vi "Diagnostics.Main.vi"(8 "error in (no error)":errorcluster, 11 "State Variables":T1={"TCP Refs"={"Connection List"=refnum, "listener ID"=refnum}, "Stop"=refnum, "Top VI"=refnum, "Parameters"={"Properties"={"Name"="", "CAN"={"CAN Interface"=enum."CAN0", "Baud Rate"=0, "Diagnostic Protocol"=enum."GMLAN", "Transport Protocol"=enum."ISO TP - Normal Mode", "Transmit ID"=0, "Receive ID"=0, "Transmit Extension"=0, "Receive Extension"=0, "Receive UUDT ID"=0, "Enable Stream"=TRUE, "VW TP Channel ID"=0, "Security"={"Source DLL Path"=path "", "Security Level"=1, "Target DLL Path"=path ""}, "Fill Frame"=FALSE, "Fill Byte"=255, "Termination"=FALSE}, "986x"={"Enable"=FALSE, "RIO Device"=0, "Bitfile"=path ""}, "Reads"=[], "Frames Lookup"=variant, "Writes"=[], "DPIDs"=[], "DPID Lookup"=variant, "DTC descriptor"={"DTC Byte Length"=2, "Status Byte Length"=1, "Add Data Byte Length"=1, "Byte Order"=enum."Motorola"}}, "ChanRefs"={"ToVS.Reads"={"Name"="", "Write to VS Engine FIFO"=refnum, "Pairs"={"Refs"=[], "Values"=[]}}, "ToVS.DTCs"={"Name"="", "Write to VS Engine FIFO"=refnum, "Pairs"={"Refs"=[], "Values"=[]}}, "ToVS.DTCCount"={"Name"="", "Write to VS Engine FIFO"=refnum, "Pairs"={"Refs"=[], "Values"=[]}}, "ToVS.Status"={"Name"="", "Write to VS Engine FIFO"=refnum, "Pairs"={"Refs"=[], "Values"=[]}}, "FromVS.Writes"={"Name"="", "Read from VS Engine FIFO"=refnum, "Pairs"={"Refs"=[], "Values"=[]}}, "Cmds"={"Name"="", "Write to VS Engine FIFO"=refnum, "Read from VS Engine FIFO"=refnum, "Pairs"={"Chan Refs"=[], "Prev. Values"=[]}}}}, "ADCS Connection"={"Diag CAN Handle"=0, "Transport Protocol"=enum."ISO TP - Normal Mode", "Receive Address Extension"=0, "Transmit Address Extension"=0, "Receive CAN Id"=0, "Transmit CAN Id"=0, "Diag CAN Queue"=refnum, "Log Frames ?"=FALSE, "My TP Address"=0, "Other TP Address"=0, "T1"=0, "T2"=0, "T3"=0, "T4"=0, "Tx SN"=0, "Block Size"=0, "Rx SN"=0, "VW TP Initialized?"=FALSE, "Tx block no"=0, "baud rate"=0, "Interface"="", "Channel Diag CAN Handle"=0, "UDP Connection ID"=refnum, "TCP Connection ID"=refnum, "Target IP Addr"=0, "Source Address"=0, "Target Address"=0, "Send Header NACK?"=FALSE, "DLL Handle"=0, "NAD"=0, "Time Stamp read first"=0.0, "Time Stamp read last"=0.0, "Time Stamp write first"=0.0, "Time Stamp write last"=0.0, "Time Stamp write"=0.0, "Time Stamp read"=0.0}, "XNET References"={"Database"="", "GMLAN DPID Session"="", "Cluster"=""}, "BufferedCmds"=refnum, "XNETEngine (GMLAN)"=refnum} {"Parameters"."ChanRefs"."Cmds"."Pairs"."Chan Refs" format="%.0x"; "Parameters"."ChanRefs"."ToVS.Status"."Pairs"."Refs" format="%.0x"; "Parameters"."ChanRefs"."ToVS.DTCCount"."Pairs"."Refs" format="%.0x"; "Parameters"."ChanRefs"."ToVS.DTCs"."Pairs"."Refs" format="%.0x"; "Parameters"."ChanRefs"."ToVS.Reads"."Pairs"."Refs" format="%.0x"; "Parameters"."Properties"."Writes"."Signals"."Byte Order" items=["Little Endian", "Big Endian"]; "Parameters"."Properties"."Writes"."Signals"."Data Type" items=["Signed", "Unsigned", "IEEE Float"]; "Parameters"."Properties"."CAN"."Fill Byte" format="%.0x"; "Parameters"."Properties"."CAN"."VW TP Channel ID" format="%.0x"; "Parameters"."Properties"."CAN"."Receive UUDT ID" format="%.0x"; "Parameters"."Properties"."CAN"."Receive Extension" format="%.0x"; "Parameters"."Properties"."CAN"."Transmit Extension" format="%.0x"; "Parameters"."Properties"."CAN"."Receive ID" format="%.0x"; "Parameters"."Properties"."CAN"."Transmit ID" format="%.0x"; "Parameters"."Properties"."Reads"."Signals"."Byte Order" items=["Little Endian", "Big Endian"]; "Parameters"."Properties"."Reads"."Signals"."Data Type" items=["Signed", "Unsigned", "IEEE Float"]}) -> (0 "error out":errorcluster)   [LabVIEW 2015, in "Diagnostics Addon Engine.lvlib"]
uses:
  Diagnostics Addon Engine.lvlib
  Types/Diagnostics.State.ctl
  Types/TCP.Refs.ctl
  STM/STM Lookup Table Ref.ctl
  Stop FG/Stop Global Ref.ctl
  Types/Engine.State.ctl
  Shared/Types/SysDef.Compile.Properties.ctl
  Shared/Types/CAN.ctl
  Shared/Types/CAN.Interface.ctl
  Shared/Types/Protocol.ctl
  Shared/Types/Transport.ctl
  Shared/Types/Security.ctl
  Shared/Types/986x.ctl
  Shared/Types/Frame.Compile.ctl
  Shared/Types/Type.ctl
  Shared/Types/Signal.ctl
  Shared/Types/DPID.ctl
  Shared/Types/DPID.Rate.ctl
  Shared/Types/DTCDescriptor.ctl
  Types/Engine.Refs.ctl
  Inline Async API/Controls/Write To VS Engine.ctl
  <vilib>/NI Veristand/Custom Device API/Data Reference.ctl
  Inline Async API/Controls/Read From VS Engine.ctl
  <vilib>/NI Veristand/Custom Device API/Block Data Reference.ctl
  Inline Async API/Controls/ReadWrite Data.ctl
  <vilib>/Automotive Diagnostic Command Set/Diagnostic Transport.llb/Diag Reference.ctl
  <vilib>/Automotive Diagnostic Command Set/Diagnostic Transport.llb/Transport Protocol Selector.ctl
  <vilib>/Automotive Diagnostic Command Set/Diagnostic Transport.llb/Diag CAN Frame Log.ctl
  Types/XNET.Refs.ctl
  <vilib>/NI/AMC/Message Queue.ctl
  <vilib>/NI/AMC/Message.ctl
  <vilib>/NI/Tools/Keyed Array/KeyedArray.ctl
  Stop FG/Global Stop Actions.vi
  Signals.Scale.EU.vi
  Frame.Build.Raw.vi
  <vilib>/NI/AMC/Send Local Message.vi
  GMLAN/Utilities/Convert Data to DTCs.vi
  DTCs.List.Update.vi
  <vilib>/NI/AMC/Read Next Message.vi
  GMLAN/_SubVIs/ReadDiagnosticInformation_ByStatus.vi
  Status.Set.vi
  GMLAN/_SubVIs/ReadDiagnosticInformation_sendOnChangeDTCCount.vi
  GMLAN/_SubVIs/ReadDiagnosticInformation_readStatusOfDTCByDTCNumber.vi
  GMLAN/_SubVIs/ReadFailureRecordData_readFailureRecordParameters.vi
  GMLAN/GMLAN DynamicallyDefineMessage.vi
  GMLAN/GMLAN ReadDataByPacketIdentifier.vi
  Signals.Scale.Raw.vi
  GMLAN/GMLAN DeviceControl.vi
  GMLAN/GMLAN TesterPresent.vi
  GMLAN/GMLAN InitiateDiagnosticOperation.vi
  GMLAN/GMLAN DisableNormalCommunication.vi
  GMLAN/GMLAN ReturnToNormalMode.vi
  ADCS.UnlockECUSecurity.vi
  <vilib>/NI/Tools/Keyed Array/Index.vi
  GMLAN/GMLAN ClearDiagnosticInformation.vi
  GMLAN/GMLAN ReadDataByParameterIdentifier.vi
  GMLAN/GMLAN ReadDataByIdentifier.vi
  Frames.Lookup.Size.Get.vi
  ADCS.TesterPresent.vi
  <vilib>/NI/AMC/Create Single Message.vi
  <vilib>/NI/AMC/Update Message Routing Info.vi
  GMLAN/Utilities/Convert Raw Data to DTCs.vi
  <vilib>/NI/AMC/Read Termination Message.vi
  <vilib>/Utility/error.llb/Clear Errors.vi
  ADCS.Get.ErrorByte.vi
  GMLAN/Utilities/GMLAN Service Broadcast.vi
  Security.DLL
  GMLAN/GMLAN SecurityAccess.vi
  GMLAN/_SubVIs/SecurityAccess_sendKey.vi
  GMLAN/_SubVIs/SecurityAccess_requestSeed.vi
  <vilib>/NI/Tools/Keyed Array/Map String.vi
  <vilib>/NI/Tools/String/Get Case Matching.vi
  Error Handling API/SubVIs/Report Error to Process.vi
  <vilib>/NI/AMC/Send Message.vi
  <vilib>/Automotive Diagnostic Command Set/Diagnostic Protocols.llb/Convert to Phys.vi
  <vilib>/xnet/xnet.llb/XNET Convert.vi
  <vilib>/xnet/xnet.llb/XNET Convert (Frame Raw to Signal).vi
  ID.Convert.Raw.vi
  <vilib>/NI Veristand/Custom Device Tools/Custom Device Utility Library/NI VeriStand - Print Debug String.vi
  <vilib>/xnet/xnet.llb/XNET Read.vi
  <vilib>/xnet/xnet.llb/XNET Read (Frame CAN).vi
  Shared/SubVIs/Constants.vi
  <vilib>/NI/AMC/Globals.vi
  <vilib>/Automotive Diagnostic Command Set/Diagnostic Protocols.llb/UDS TesterPresent.vi
  <vilib>/Automotive Diagnostic Command Set/Diagnostic Transport.llb/Apply Success Failure Error.vi
  <vilib>/Automotive Diagnostic Command Set/Diagnostic Transport.llb/Diagnostic Service.vi
  <vilib>/Automotive Diagnostic Command Set/Diagnostic Transport.llb/Apply Diagnostic Error.vi
  <vilib>/Automotive Diagnostic Command Set/Diagnostic Transport.llb/Diagnostic Response Recv.vi
  <vilib>/Automotive Diagnostic Command Set/Diagnostic Transport.llb/Diagnostic Service Send.vi
  <vilib>/Automotive Diagnostic Command Set/Diagnostic Transport.llb/Diag Globals.vi
  <vilib>/Automotive Diagnostic Command Set/Diagnostic Protocols.llb/TesterPresent.vi
  <vilib>/Automotive Diagnostic Command Set/Diagnostic Protocols.llb/UDS RoutineControl.vi
  <vilib>/Automotive Diagnostic Command Set/Diagnostic Protocols.llb/StopRoutineByLocalIdentifier.vi
  <vilib>/xnet/xnet.llb/XNET Convert (Signal to Frame Raw).vi
  <vilib>/Automotive Diagnostic Command Set/Diagnostic Protocols.llb/RequestRoutineResultsByLocalIdentifier.vi
  <vilib>/Automotive Diagnostic Command Set/Diagnostic Protocols.llb/StartRoutineByLocalIdentifier.vi
  <vilib>/Automotive Diagnostic Command Set/Diagnostic Protocols.llb/UDS InputOutputControlByIdentifier.vi
  <vilib>/Automotive Diagnostic Command Set/Diagnostic Protocols.llb/InputOutputControlByLocalIdentifier.vi
  <vilib>/Automotive Diagnostic Command Set/Diagnostic Protocols.llb/UDS WriteMemoryByAddress.vi
  <vilib>/Automotive Diagnostic Command Set/Diagnostic Protocols.llb/UDS06 WriteMemoryByAddress.vi
  <vilib>/Automotive Diagnostic Command Set/Diagnostic Protocols.llb/WriteMemoryByAddress.vi
  <vilib>/Automotive Diagnostic Command Set/Diagnostic Protocols.llb/UDS ReadMemoryByAddress.vi
  <vilib>/Automotive Diagnostic Command Set/Diagnostic Protocols.llb/UDS06 ReadMemoryByAddress.vi
  <vilib>/Automotive Diagnostic Command Set/Diagnostic Protocols.llb/ReadMemoryByAddress.vi
  <vilib>/Automotive Diagnostic Command Set/Diagnostic Protocols.llb/UDS ECUReset.vi
  <vilib>/Automotive Diagnostic Command Set/Diagnostic Protocols.llb/ECUReset.vi
  <vilib>/Automotive Diagnostic Command Set/Diagnostic Protocols.llb/ControlDTCSetting.vi
  <vilib>/Automotive Diagnostic Command Set/Diagnostic Protocols.llb/UDS ControlDTCSetting.vi
  <vilib>/Automotive Diagnostic Command Set/Diagnostic Protocols.llb/UDS WriteDataByIdentifier.vi
  <vilib>/Automotive Diagnostic Command Set/Diagnostic Protocols.llb/WriteDataByLocalIdentifier.vi
  <vilib>/Automotive Diagnostic Command Set/Diagnostic Protocols.llb/UDS ReadDataByIdentifier.vi
  <vilib>/Automotive Diagnostic Command Set/Diagnostic Protocols.llb/ReadDataByLocalIdentifier.vi
  <vilib>/Automotive Diagnostic Command Set/Diagnostic Protocols.llb/UDS ClearDiagnosticInformation.vi
  <vilib>/Automotive Diagnostic Command Set/Diagnostic Protocols.llb/ClearDiagnosticInformation.vi
  <vilib>/Automotive Diagnostic Command Set/Diagnostic Protocols.llb/ReadDTCByStatus.vi
  <vilib>/Automotive Diagnostic Command Set/Diagnostic Protocols.llb/ReadStatusOfDTC.vi
  <vilib>/Automotive Diagnostic Command Set/Diagnostic Protocols.llb/UDS ReportDTCByStatusMask.vi
  <vilib>/Automotive Diagnostic Command Set/Diagnostic Protocols.llb/UDS ReportSeverityInformationOfDTC.vi
  <vilib>/Automotive Diagnostic Command Set/Diagnostic Protocols.llb/UDS ReportDTCBySeverityMaskRecord.vi
  <vilib>/Automotive Diagnostic Command Set/Diagnostic Protocols.llb/SendKey.vi
  <vilib>/Automotive Diagnostic Command Set/Diagnostic Protocols.llb/UDS SendKey.vi
  <vilib>/Automotive Diagnostic Command Set/Diagnostic Protocols.llb/RequestSeed.vi
  <vilib>/Automotive Diagnostic Command Set/Diagnostic Protocols.llb/UDS RequestSeed.vi
  <vilib>/Automotive Diagnostic Command Set/Diagnostic Protocols.llb/EnableNormalMessageTransmission.vi
  <vilib>/Automotive Diagnostic Command Set/Diagnostic Protocols.llb/UDS CommunicationControl.vi
  <vilib>/Automotive Diagnostic Command Set/Diagnostic Protocols.llb/DisableNormalMessageTransmission.vi
  <vilib>/Automotive Diagnostic Command Set/Diagnostic Protocols.llb/UDS DiagnosticSessionControl.vi
  <vilib>/Automotive Diagnostic Command Set/Diagnostic Protocols.llb/StopDiagnosticSession.vi
  <vilib>/Automotive Diagnostic Command Set/Diagnostic Protocols.llb/StartDiagnosticSession.vi
  <vilib>/Automotive Diagnostic Command Set/Diagnostic Transport.llb/Diag Set Property.vi
  <vilib>/Automotive Diagnostic Command Set/Diagnostic Transport.llb/Diag Get Property.vi
  DPIDs.IDs.Sort.vi
  Shared/Diagnostics Addon Shared.lvlib
  <vilib>/NI Veristand/Custom Device API/Custom Device API.lvlib
  <vilib>/NI/Tools/Keyed Array/Tools_KeyedArray.lvlib
  <vilib>/NI/AMC/AMC.lvlib
  <vilib>/addons/Automotive Diagnostic Command Set/NI_Automotive Diagnostic Command Set.lvlib
  Inline Async API/Inline Async API.lvlib
  Stop FG/Stop FG.lvlib
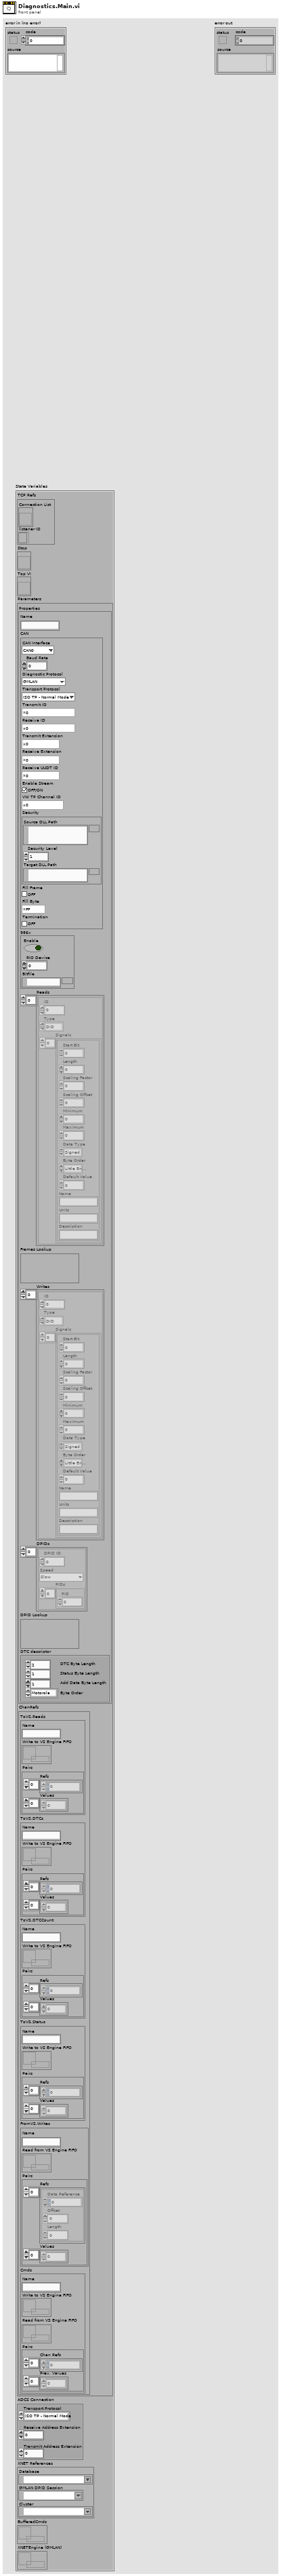
[diagram p1: front panel]
types:
  T1 = typedef "Diagnostics Addon Engine.lvlib/Diagnostics.State.ctl" = cluster{"TCP Refs":T2, "Stop":T4, "Top VI":refnum<vi>, "Parameters":T5, "ADCS Connection":T25, "XNET References":T27, "BufferedCmds":T28, "XNETEngine (GMLAN)":T28}
  T2 = typedef "Diagnostics Addon Engine.lvlib/TCP.Refs.ctl" = cluster{"Connection List":T3, "listener ID":refnum<k5>}
  T3 = typedef "Diagnostics Addon Engine.lvlib/STM Lookup Table Ref.ctl" = refnum<vi>
  T4 = typedef "Diagnostics Addon Engine.lvlib/Stop FG.lvlib/Stop Global Ref.ctl" = refnum<vi>
  T5 = typedef "Diagnostics Addon Engine.lvlib/Engine.State.ctl" = cluster{"Properties":T6, "ChanRefs":T19}
  T6 = typedef "Diagnostics Addon Shared.lvlib/SysDef.Compile.Properties.ctl" = cluster{"Name":string, "CAN":T7, "986x":T12, "Reads":T13[], "Frames Lookup":variant, "Writes":T13[], "DPIDs":T16[], "DPID Lookup":variant, "DTC descriptor":T18}
  T7 = typedef "Diagnostics Addon Shared.lvlib/CAN.ctl" = cluster{"CAN Interface":T8, "Baud Rate":u32, "Diagnostic Protocol":T9, "Transport Protocol":T10, "Transmit ID":u32, "Receive ID":u32, "Transmit Extension":u8, "Receive Extension":u8, "Receive UUDT ID":u32, "Enable Stream":bool, "VW TP Channel ID":u32, "Security":T11, "Fill Frame":bool, "Fill Byte":u8, "Termination":bool}
  T8 = typedef "Diagnostics Addon Shared.lvlib/CAN.Interface.ctl" = enum16{"CAN0", "CAN1", "CAN2", "CAN3", "CAN4", "CAN5", "CAN6", "CAN7", "CAN8", "CAN9", "CAN10", "CAN11", "CAN12", "CAN13", "CAN14", "CAN15", "CAN16", "CAN17", "CAN18", "CAN19", "CAN20", "CAN21", "CAN22", "CAN23", "CAN24", "CAN25", "CAN26", "CAN27", "CAN28", "CAN29", "CAN30", "CAN31", "CAN32", "CAN33", "CAN34", "CAN35", "CAN36", "CAN37", "CAN38", "CAN39", "CAN40", "CAN41", "CAN42", "CAN43", "CAN44", "CAN45", "CAN46", "CAN47", "CAN48", "CAN49", "CAN50", "CAN51", "CAN52", "CAN53", "CAN54", "CAN55", "CAN56", "CAN57", "CAN58", "CAN59", "CAN60", "CAN61", "CAN62", "CAN63", "CAN 256 (Virtual)", "CAN 257 (Virtual)"}
  T9 = typedef "Diagnostics Addon Shared.lvlib/Protocol.ctl" = enum16{"GMLAN", "KWP-2000", "UDS"}
  T10 = typedef "Diagnostics Addon Shared.lvlib/Transport.ctl" = enum16{"ISO TP - Normal Mode", "ISO TP - Mixed Mode", "VW TP 2.0", "Diagnostics on IP"}
  T11 = typedef "Diagnostics Addon Shared.lvlib/Security.ctl" = cluster{"Source DLL Path":path, "Security Level":u8, "Target DLL Path":path}
  T12 = typedef "Diagnostics Addon Shared.lvlib/986x.ctl" = cluster{"Enable":bool, "RIO Device":u16, "Bitfile":path}
  T13 = typedef "Diagnostics Addon Shared.lvlib/Frame.Compile.ctl" = cluster{"ID":u32, "Type":T14, "Signals":T15[]}
  T14 = typedef "Diagnostics Addon Shared.lvlib/Type.ctl" = enum16{"DID", "CDID", "PID", "CPID", "Read Memory", "Write Memory", "DTC Control", "IO Cmd", "IO Resp", "Routine Start Cmd", "Routine Start Resp", "Routine Request Cmd", "Routine Request Resp", "Routine Stop Cmd", "Routine Stop Resp"}
  T15 = typedef "Diagnostics Addon Shared.lvlib/Signal.ctl" = cluster{"Start Bit":u8, "Length":u8, "Scaling Factor":dbl, "Scaling Offset":dbl, "Minimum":dbl, "Maximum":dbl, "Data Type":u32, "Byte Order":u32, "Default Value":dbl, "Name":string, "Units":string, "Description":string}
  T16 = typedef "Diagnostics Addon Shared.lvlib/DPID.ctl" = cluster{"DPID ID":u8, "Speed":T17, "PIDs":u16[]}
  T17 = typedef "Diagnostics Addon Shared.lvlib/DPID.Rate.ctl" = enum16{"Slow", "Medium", "Fast"}
  T18 = typedef "Diagnostics Addon Shared.lvlib/DTCDescriptor.ctl" = cluster{"DTC Byte Length":i32, "Status Byte Length":i32, "Add Data Byte Length":i32, "Byte Order":enum16{"Motorola", "Intel"}}
  T19 = typedef "Diagnostics Addon Engine.lvlib/Engine.Refs.ctl" = cluster{"ToVS.Reads":T20, "ToVS.DTCs":T20, "ToVS.DTCCount":T20, "ToVS.Status":T20, "FromVS.Writes":T22, "Cmds":T24}
  T20 = typedef "Diagnostics Addon Engine.lvlib/Inline Async API.lvlib/Write To VS Engine.ctl" = cluster{"Name":string, "Write to VS Engine FIFO":refnum<k33>, "Pairs":cluster{"Refs":T21[], "Values":dbl[]}}
  T21 = typedef "Custom Device API.lvlib/Data Reference.ctl" = i32
  T22 = typedef "Diagnostics Addon Engine.lvlib/Inline Async API.lvlib/Read From VS Engine.ctl" = cluster{"Name":string, "Read from VS Engine FIFO":refnum<k33>, "Pairs":cluster{"Refs":T23[], "Values":dbl[]}}
  T23 = typedef "Custom Device API.lvlib/Block Data Reference.ctl" = cluster{"Data Reference":T21, "Offset":u64, "Length":u64}
  T24 = typedef "Diagnostics Addon Engine.lvlib/Inline Async API.lvlib/ReadWrite Data.ctl" = cluster{"Name":string, "Write to VS Engine FIFO":refnum<k33>, "Read from VS Engine FIFO":refnum<k33>, "Pairs":cluster{"Chan Refs":T21[], "Prev. Values":dbl[]}}
  T25 = typedef "NI_Automotive Diagnostic Command Set.lvlib/Diag Reference.ctl" = cluster{"Diag CAN Handle":u32, "Transport Protocol":T26, "Receive Address Extension":u8, "Transmit Address Extension":u8, "Receive CAN Id":u32, "Transmit CAN Id":u32, "Diag CAN Queue":refnum<queue>, "Log Frames ?":bool, "My TP Address":u8, "Other TP Address":u8, "T1":u16, "T2":u16, "T3":u16, "T4":u16, "Tx SN":u8, "Block Size":u8, "Rx SN":u8, "VW TP Initialized?":bool, "Tx block no":u8, "baud rate":u32, "Interface":string, "Channel Diag CAN Handle":u32, "UDP Connection ID":refnum<k16>, "TCP Connection ID":refnum<k5>, "Target IP Addr":u32, "Source Address":u16, "Target Address":u16, "Send Header NACK?":bool, "DLL Handle":u32, "NAD":u8, "Time Stamp read first":dbl, "Time Stamp read last":dbl, "Time Stamp write first":dbl, "Time Stamp write last":dbl, "Time Stamp write":dbl, "Time Stamp read":dbl}
  T26 = typedef "NI_Automotive Diagnostic Command Set.lvlib/Transport Protocol Selector.ctl" = enum16{"ISO TP - Normal Mode", "ISO TP - Mixed Mode", "VW TP 2.0", "Diagnostics on IP", "ISO TP LIN"}
  T27 = typedef "Diagnostics Addon Engine.lvlib/XNET.Refs.ctl" = cluster{"Database":refnum<k21>, "GMLAN DPID Session":refnum<k21>, "Cluster":refnum<k21>}
  T28 = typedef "AMC.lvlib/Message Queue.ctl" = refnum<queue>
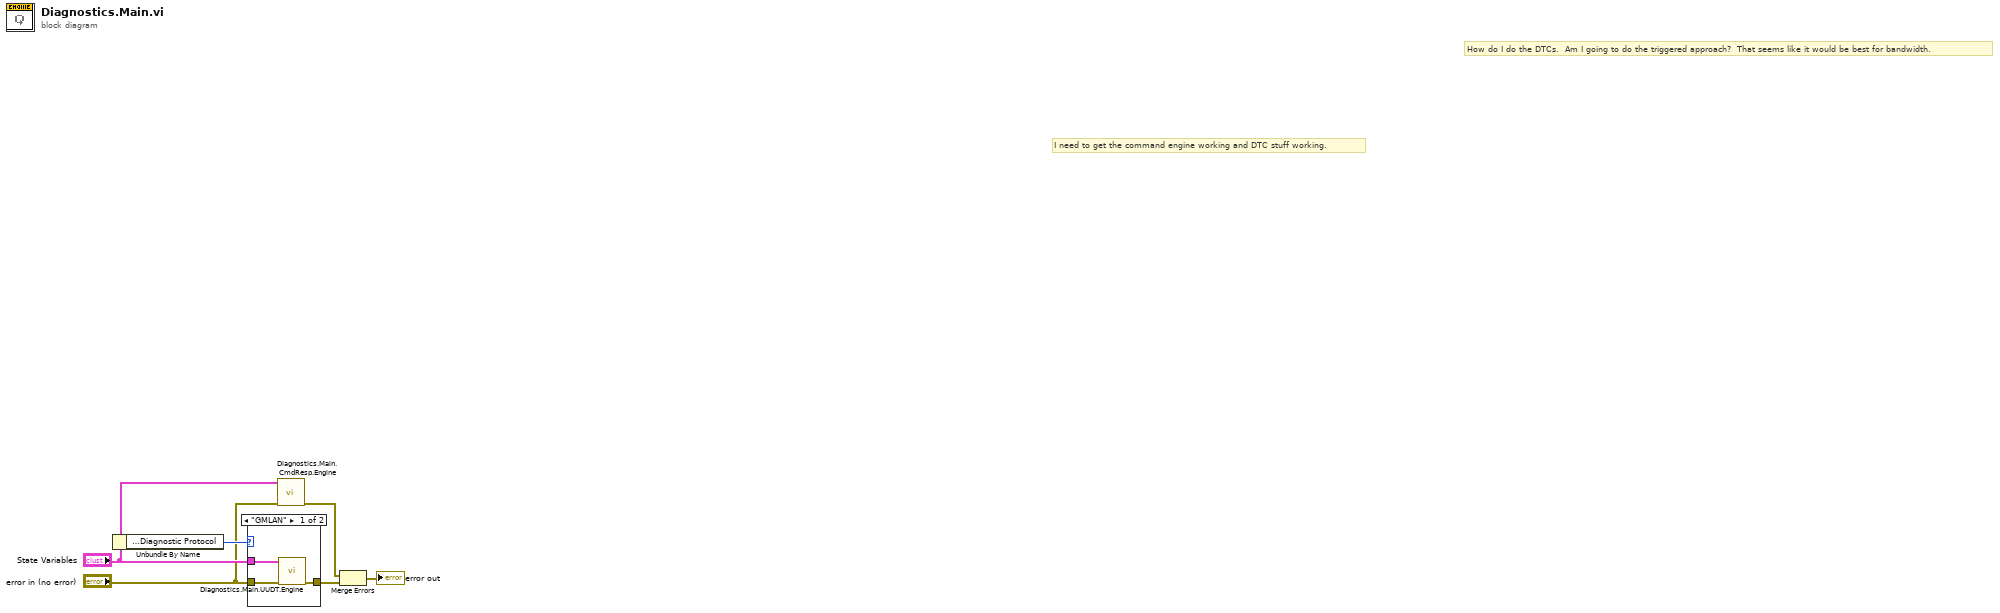
[diagram p0: block diagram]
diagram:
  # "How do I do the DTCs.  Am I going to do the triggered approach?  That seems like it would be best for bandwidth."
  # "I need to get the command engine working and DTC stuff working."
  n1 = Unbundle By Name("State Variables") -> ("Parameters.Properties.CAN.Diagnostic Protocol"=w6:T9)
  n2 = case shown="\"GMLAN\"" w6 {
    tunnel: "State Variables" -> [w9 _]
    tunnel: [w7 w10] -> w4
    tunnel: "error in (no error)" -> [w8 w10]
    frame "GMLAN" {
      n3 = call "Diagnostics.Main.UUDT.Engine.vi"("error in (no error)"=w8, "State Variables"=w9) -> ("error out"=w7:errorcluster)  [unwired: 9 in]
    }
    frame "KWP-2000", "UDS" {
    }
  }
  n4 = call "Diagnostics.Main.CmdResp.Engine.vi"("error in (no error)"="error in (no error)", "State Variables"="State Variables") -> ("error out"=w3:errorcluster)  [unwired: 9 in]
  n5 = Merge Errors(w3, w4) -> (→"error out":errorcluster)
